vi "Client Spawner.vi"() -> ()   [LabVIEW 2011]
panel:
  in  "# to spawn":i32=2
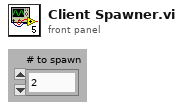
[diagram p1: front panel]
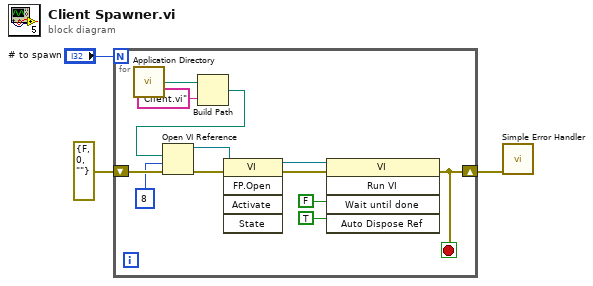
[diagram p0: block diagram]
diagram:
  n1 = for {
    N: "# to spawn" -> [_]
    shift-right: [w11] -> w1
    shift-left: errorcluster {"status"=FALSE, "code"=0, "source"=""} ("error out") -> [w10]
    stop <- w11 stop-if-true
    n2 = call <vilib>:"Application Directory.vi"() -> ("Application Directory"=w7:path)
    n3 = Build Path(base path=w7, name or relative path="Client.vi") -> (appended path=w5:path)
    n4 = Open VI Reference(vi path=w5, options=8, error in (no error)=w10) -> (vi reference=w8:refnum<vi>, error out=w9:errorcluster)  [unwired: 3 in]
    n5 = invoke class="VI" method="FP.Open"(reference=w8, error in=w9) -> (reference out=w15:refnum<vi>, error out=w14:errorcluster)  [unwired: 3 in, 3 out]
    n6 = invoke class="VI" method="Run VI"(reference=w15, error in=w14, "Wait until done"=FALSE ("Wait Until Done"), "Auto Dispose Ref"=TRUE ("Auto Dispose Reference")) -> (error out=w11:errorcluster)  [unwired: 1 in, 4 out]
  }
  n7 = call <vilib>:"Simple Error Handler.vi"("error in (no error)"=w1) -> ()  [unwired: 4 in, 5 out]
